vi "PPSU MS Init.vi"(8 "Error in":errorcluster, 11 "Device information arrayR":string[](array[string])) -> (0 "Fehler (Ausgang)":errorcluster caption="Error out", 3 "Device information out":string[](array[string]))   [LabVIEW 2022 SP3]
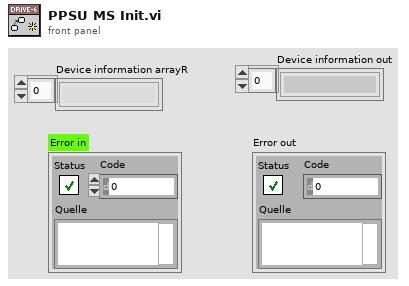
[diagram p1: front panel]
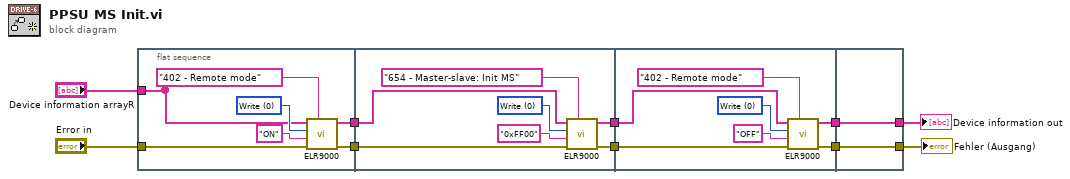
[diagram p0: block diagram]
diagram:
  n1 = flat-sequence {
    tunnel: "Error in" -> [w17]
    tunnel: [w11] -> _
    tunnel: [w13] -> w10
    tunnel: [w12] -> w9
    tunnel: "Device information arrayR" -> [w11]
    tunnel: w10 -> [w24]
    tunnel: w9 -> [w23]
    tunnel: [w19] -> w8
    tunnel: [w18] -> w7
    tunnel: w8 -> [w31]
    tunnel: w7 -> [w30]
    tunnel: [w26] -> w6
    tunnel: [w25] -> w5
    tunnel: w6 -> [w32]
    tunnel: w5 -> [w33]
    tunnel: [w33] -> w3
    tunnel: [w32] -> w2
    frame #0 {
      w15 = u8 0 items=["Write", "Read"] ("Access")
      n2 = call <vilib>:"ELR9000.vi"("Command list"="402 - Remote mode", "Error in"=w17, "Value"="ON", "Access"=w15, "Device information in"=w11) -> ("Error out"=w12:errorcluster, "Device information out"=w13:string[])  [unwired: 1 in, 2 out]
    }
    frame #1 {
      w21 = u8 0 items=["Write", "Read"] ("Access")
      n3 = call <vilib>:"ELR9000.vi"("Command list"="654 - Master-slave: Init MS", "Error in"=w23, "Value"="0xFF00", "Access"=w21, "Device information in"=w24) -> ("Error out"=w19:errorcluster, "Device information out"=w18:string[])  [unwired: 1 in, 2 out]
    }
    frame #2 {
      w28 = u8 0 items=["Write", "Read"] ("Access")
      n4 = call <vilib>:"ELR9000.vi"("Command list"="402 - Remote mode", "Error in"=w31, "Value"="OFF", "Access"=w28, "Device information in"=w30) -> ("Error out"=w26:errorcluster, "Device information out"=w25:string[])  [unwired: 1 in, 2 out]
    }
    frame #3 {
    }
  }
  "Device information out" <- w3
  "Fehler (Ausgang)" <- w2
